vi "GlobalCameraHandle.vi"() -> ()   [LabVIEW 2011]
panel:
  in  "CameraHandle":dbl
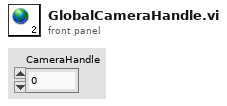
[diagram p1: front panel]
diagram:
